vi "LibXML_GetStringLength.vi"(4 "error in":errorcluster, 6 "string pointer":u32) -> (0 "error out":errorcluster, 3 "string length":i32)   [LabVIEW 2019, in "Tools.lvlib" / "LibXML.lvlib"]
uses:
  LibXML.lvlib
  dll/lXMLwrap.dll
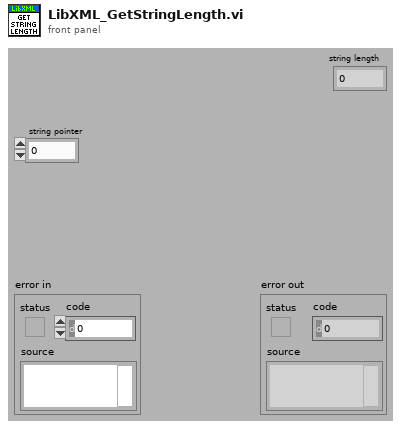
[diagram p1: front panel]
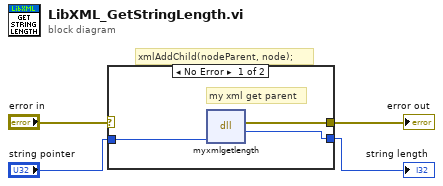
[diagram p0: block diagram]
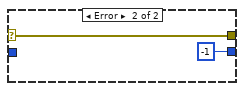
[diagram p2: hidden frame]
diagram:
  # "xmlAddChild(nodeParent, node);"
  n1 = case shown="No Error" "error in" {
    selector: "error in" -> [_ w9]
    tunnel: [w5 w9] -> w3
    tunnel: "string pointer" -> [w7 _]
    tunnel: [w6 -1 ("return type")] -> w1
    frame No Error {
      # "my xml get parent"
      n2 = dll-call lib="C:/Projects/_Prywatne/MyCIT/Framework/Tools/XML/LibXML/dll/lXMLwrap.dll" fn="myxmlgetlength"("node"=w7) -> (error out=w5:errorcluster, "return type"=w6:i32)  [unwired: 4 in, 1 out]
    }
    frame Error {
    }
  }
  "error out" <- w3
  "string length" <- w1
